vi "ColorDialog.vi"(8 "错误输入（无错误）":errorcluster, 11 "FullOpen":bool) -> (0 "错误输出":errorcluster, 1 "ShowDialog":i32(ring) items=["None", "OK", "Cancel", "Abort", "Retry", "Ignore", "Yes", "No"], 3 "Color":u32(colorbox) caption="颜色")   [LabVIEW 2012]
uses:
  System.Windows.Forms
  System.Drawing
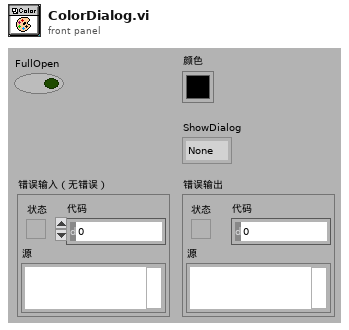
[diagram p1: front panel]
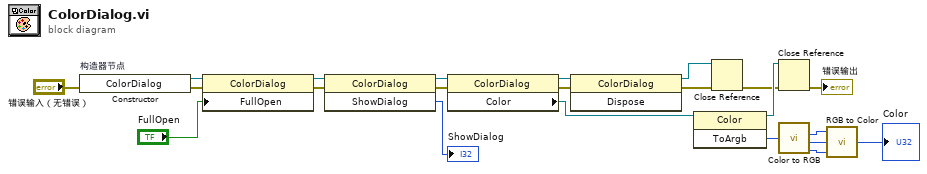
[diagram p0: block diagram]
diagram:
  n1 = constructor on="构造器节点" class="ColorDialog"(error in="错误输入（无错误）") -> (reference out=w22:refnum<k24>, error out=w21:errorcluster)  [unwired: 2 in, 1 out]
  n2 = property class="ColorDialog"(reference=w22, error in=w21, "FullOpen"="FullOpen") -> (reference out=w19:refnum<k24>, error out=w20:errorcluster)
  n3 = invoke class="ColorDialog" method="ShowDialog"(reference=w19, error in=w20) -> (reference out=w14:refnum<k24>, error out=w15:errorcluster, "ShowDialog"=→"ShowDialog":i32)  [unwired: 1 in]
  n4 = property class="ColorDialog"(reference=w14, error in=w15) -> (reference out=w13:refnum<k24>, error out=w12:errorcluster, "Color"=w11:refnum<k24>)
  n5 = invoke class="ColorDialog" method="Dispose"(reference=w13, error in=w12) -> (reference out=w17:refnum<k24>, error out=w16:errorcluster)  [unwired: 1 in, 1 out]
  n6 = invoke class="Color" method="ToArgb"(reference=w11) -> (reference out=w6:refnum<k24>, "ToArgb"=w1:i32)  [unwired: 2 in, 1 out]
  n7 = Close Reference(reference=w17, error in (no error)=w16) -> (error out=w5:errorcluster)
  n8 = Close Reference(reference=w6, error in (no error)=w5) -> (error out=→"错误输出":errorcluster)
  n9 = call <vilib>:"Color to RGB.vi"("Color"=w1) -> ("R"=w10:u8, "G"=w9:u8, "B"=w8:u8)  [unwired: 1 out]
  n10 = call <vilib>:"RGB to Color.vi"("B"=w8, "G"=w9, "R"=w10) -> ("Color"=→"Color":u32)
